vi "SLL DE Insert Array Subset v1.vi"(8 "error in (no error)":errorcluster, 9 "New element":tag[](array[tag]), 10 "Channel index":i32, 11 "Channel Name":cluster{tag[]}[](array[cluster])) -> (0 "error out":errorcluster, 3 "Channel Name":cluster{"New element":tag[]}[](array[cluster]))   [LabVIEW 2013]
doc: "Copyright © 2005, Soliton Technologies.\nAll rights reserved."
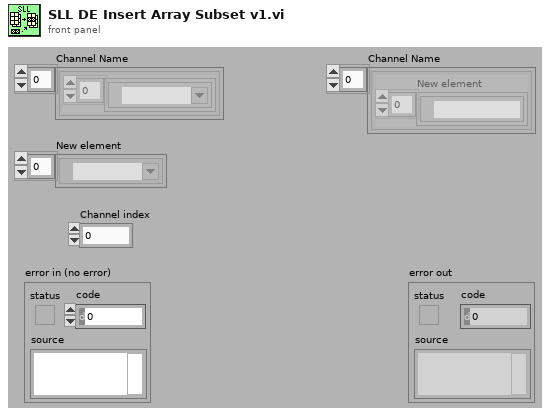
[diagram p1: front panel]
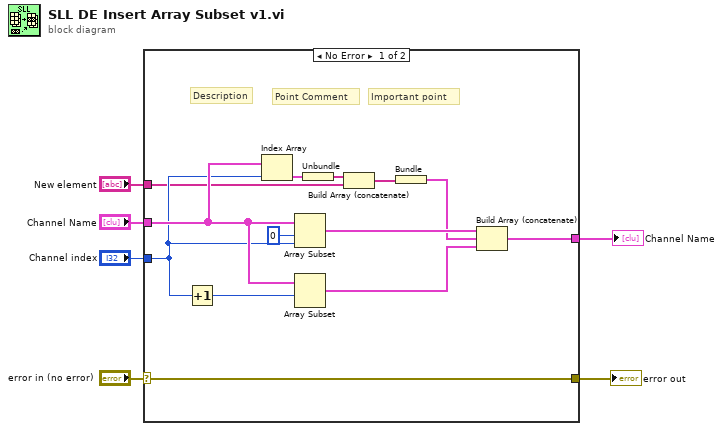
[diagram p0: block diagram]
diagram:
  n1 = case shown="No Error" "error in (no error)" {
    selector: "error in (no error)" -> [w19 w21]
    tunnel: [w19 w21] -> w5
    tunnel: "Channel Name" -> [w13 w20]
    tunnel: "Channel index" -> [w12 _]
    tunnel: "New element" -> [w9 _]
    tunnel: [w14 w20] -> w1
    frame No Error {
      # "Point Comment"
      # "Important point"
      # "Description"
      n2 = Increment(x=w12) -> (x+1=w17:i32)
      n3 = Index Array(array=w13, index=w12) -> (element=w11:cluster{tag[]})
      n4 = Array Subset(array=w13, index=0, length=w12) -> (w16:cluster{tag[]}[])
      n5 = Array Subset(array=w13, index=w17) -> (w15:cluster{tag[]}[])  [unwired: 1 in]
      n6 = Unbundle(w11) -> (w10:tag[])
      n7 = Build Array (concatenate)(w10, w9) -> (w8:tag[])
      n8 = Bundle(w8) -> (w7:cluster{tag[]})  [unwired: 1 in]
      n9 = Build Array (concatenate)(w16, w7, w15) -> (w14:cluster{tag[]}[])
    }
    frame Error {
    }
  }
  "error out" <- w5
  "Channel Name" <- w1
